vi "Unicode Picture Control Example.vi"() -> ()   [LabVIEW 2020]
doc: "This example demonstrates writing unicode text to a 2D picture control."
uses:
  Unicode/Controls/String Encoding.ctl
  Types/UTF-8 String/UTF-8 String.lvclass/UTF-8 String.ctl
  Private/Conversion/Text to UTF-8.vi
  Private/Conversion/Polymorphic VIs/Text to UTF-8 (LabVIEW String).vi
  Private/Conversion/Encoded UTF-8 String to Encoded UTF-16LE String.vi
  Unicode/SubVIs/UTF-16 Byte Swap.vi
  Private/Conversion/UTF-8 to Text.vi
  Private/Conversion/Polymorphic VIs/UTF-8 to Text (LabVIEW String).vi
  Private/Conversion/Encoded UTF-16LE String to Encoded UTF-8 String.vi
  Unicode/Prepend BOM.vi
  Unicode/SubVIs/Byte Order Marks.vi
  Unicode/Detect BOM.vi
  Unicode/Detect String Encoding.vi
  Types/UTF-8 String/UTF-8 String.lvclass
  G-Unicode.lvlib
panel:
  in  "Party Mode":bool
  in  "Stop":bool
  out "Picture":picture
  # "Instructions:\n1. Run the VI.\n2. Unicode text will be drawn to the picture control."
  # "G"
  # "-Unicode"
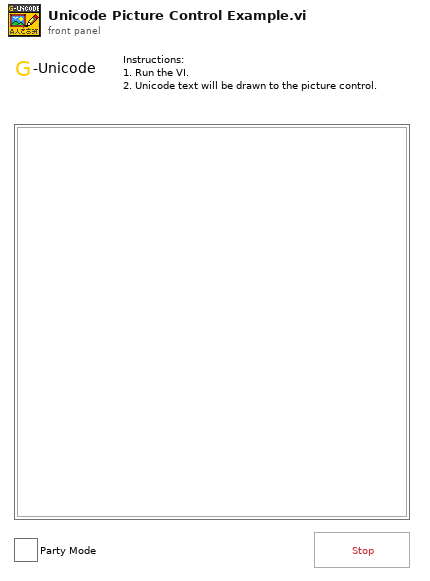
[diagram p1: front panel]
types:
  T1 = cluster{"Font Name:":string, "Size":i16, "Strikeout?":bool, "Italic?":bool, "Underline?":bool, "Outline?":bool, "Shadow?":bool, "Bold?":bool}
  T2 = typedef "G-Unicode.lvlib/String Encoding.ctl" = enum16{"ANSI", "UTF-8", "UTF-16LE", "UTF-16BE", "Unknown"}
  T3 = typedef "LVBoundsTypeDef.ctl" = cluster{"Width":u32, "Height":u32}
  T4 = cluster{"horizontal":enum16{"left", "center", "right"}, "vertical":enum16{"top", "center", "bottom"}}
  T5 = enum16{"User-specified Font", "Application Font", "System Font", "Dialog Font"}
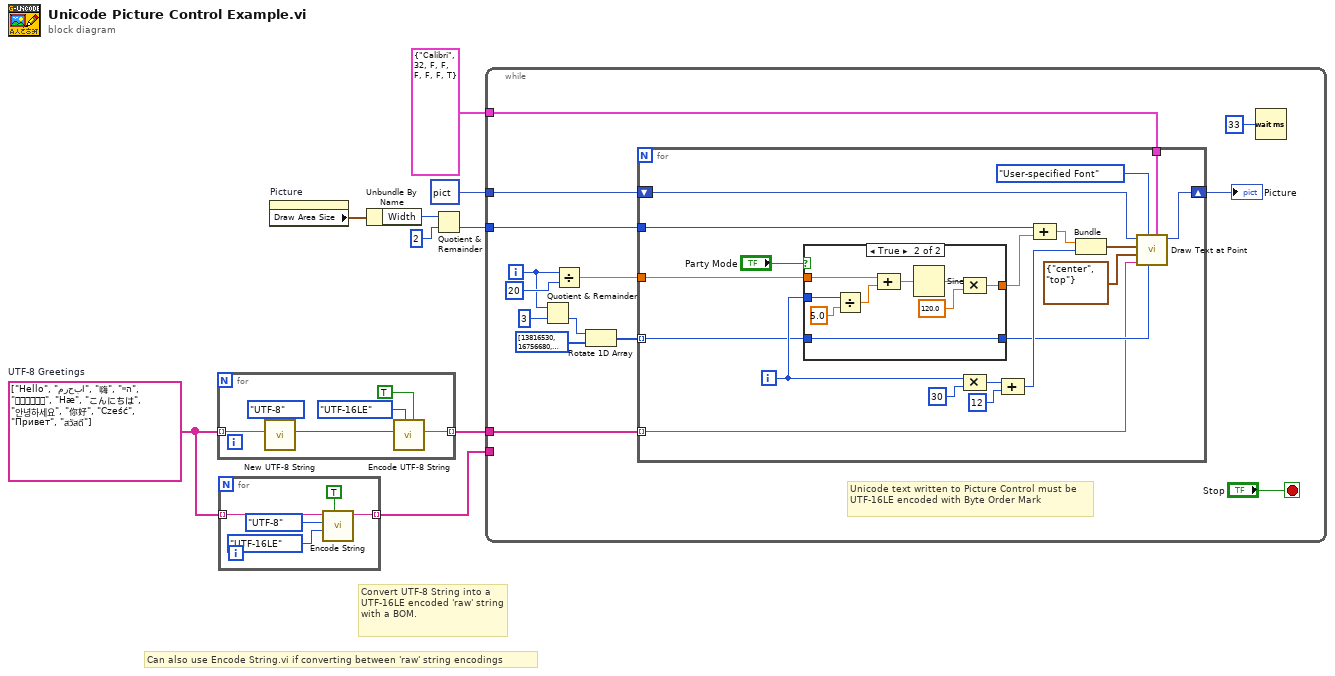
[diagram p0: block diagram]
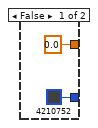
[diagram p2: hidden frame]
diagram:
  w8 = string[] ["Hello", "مرحبا", "嗨", "היי", "नमस्ते", "Hæ", "こんにちは", "안녕하세요", "你好", "Cześć", "Привет", "สวัสดี"]  # UTF-8 Greetings
  # "Convert UTF-8 String into a UTF-16LE encoded 'raw' string with a BOM."
  # "Can also use Encode String.vi if converting between 'raw' string encodings"
  n1 = for {
    tunnel: w8 -> [w15] mode=indexing
    tunnel: [w10] -> w9 mode=indexing
    n2 = call "New UTF-8 String.vi"("Input Encoding (ANSI)"=String_Encoding."UTF-8", "String"=w15) -> ("UTF-8 String"=w11:refnum<class "UTF-8 String.lvclass">)  [unwired: 8 in, 1 out]
    n3 = call "Encode UTF-8 String.vi"("Prepend BOM (F)"=TRUE, "Output Encoding (UTF-16LE)"=String_Encoding."UTF-16LE", "UTF-8 String"=w11) -> ("Encoded String"=w10:string)  [unwired: 7 in, 1 out]
  }
  n4 = for {
    tunnel: w8 -> [w20] mode=indexing
    tunnel: [w16] -> w2 mode=indexing
    n5 = call "Encode String.vi"("Prepend BOM (F)"=TRUE, "Output Encoding (UTF-16LE)"=String_Encoding."UTF-16LE", "Input Encoding (ANSI)"=String_Encoding."UTF-8", "String in"=w20) -> ("String out"=w16:string)  [unwired: 6 in, 1 out]
  }
  n6 = property on="Picture" class="Pict"() -> ("Draw Area Size"=w4:T3)  [unwired: 2 in, 2 out]
  n7 = Unbundle By Name(w4) -> ("Width"=w3:u32)
  n8 = Quotient & Remainder(x=w3, y=u32 2) -> (floor(x/y)=w6:u32)  [unwired: 1 out]
  n9 = while {
    tunnel: w9 -> [w24]
    tunnel: picture data[5B] ("new picture") -> [w34]
    tunnel: w6 -> [w31]
    tunnel: w2 -> [_]
    tunnel: T1 {"Font Name:"="Calibri", "Size"=32, "Strikeout?"=FALSE, "Italic?"=FALSE, "Underline?"=FALSE, "Outline?"=FALSE, "Shadow?"=FALSE, "Bold?"=TRUE} ("[user-specified font]") -> [w21]
    i -> [w26]
    stop <- "Stop" stop-if-true
    # "Unicode text written to Picture Control must be UTF-16LE encoded with Byte Order Mark"
    n10 = Quotient & Remainder(x=w26, y=3) -> (floor(x/y)=w23:i32)  [unwired: 1 out]
    n11 = Divide(x=w26, y=20) -> (x/y=w30:dbl)
    n12 = Rotate 1D Array(1:u32[] [13816530, 16756680, 7657454, 6371605, 0, 14942979, 16747520, 16772352, 32806, 19947, 7669639, 16711808], 2:w23) -> (0:w22:u32[])
    n13 = for {
      tunnel: w24 -> [w35] mode=indexing
      shift-right: [w52] -> w33
      shift-left: w34 -> [w53]
      tunnel: w21 -> [w50]
      tunnel: w31 -> [w39]
      tunnel: w30 -> [w42]
      tunnel: w22 -> [w36] mode=indexing
      i -> [w40]
      n14 = case shown="True" "Party Mode" {
        tunnel: [0.0 w63] -> w43
        tunnel: w42 -> [_ w62]
        tunnel: w40 -> [_ w58]
        tunnel: [u32 4210752 ("text color(black)") w56] -> w37
        tunnel: w36 -> [_ w56]
        frame False {
        }
        frame True {
          n15 = Divide(x=w58, y=5.0) -> (x/y=w59:dbl)
          n16 = Compound Arithmetic op=ADD(w62, w59) -> (w61:dbl)
          n17 = Sine(x=w61) -> (sin(x)=w64:dbl)
          n18 = Compound Arithmetic op=MULTIPLY(w64, 120.0 ("value")) -> (w63:dbl)
        }
      }
      n19 = Compound Arithmetic op=MULTIPLY(w40, 30 ("y")) -> (w41:i32)
      n20 = Compound Arithmetic op=ADD(w41, 12 ("value")) -> (w45:i32)
      n21 = Compound Arithmetic op=ADD(w39, w43) -> (w48:dbl)
      n22 = Bundle(w48, w45) -> (w44:cluster{dbl, i32})  [unwired: 1 in]
      n23 = call <vilib>:"Draw Text at Point.vi"("[user-specified font]"=w50, "text color(black)"=w37, "desired font(Application)"=T5."User-specified Font", "text"=w35, "alignment(left, top)"=T4 {"horizontal"=enum."center", "vertical"=enum."top"}, "origin"=w44, "picture"=w53) -> ("new picture"=w52:picture)  [unwired: 3 in, 1 out]
    }
    "Picture" <- w33
    n24 = Wait (ms)(milliseconds to wait=u32 33) -> ()  [unwired: 1 out]
  }
